vi "set Always On Top.vi"(8 "error in (no error)":errorcluster, 10 "Always On Top":bool, 11 "Actor in":refnum<class "Actor.lvclass">) -> (0 "error out":errorcluster, 3 "Actor out":refnum<class "Actor.lvclass">)   [LabVIEW 2015, in "Actor.lvclass"]
uses:
  Actor.lvclass
  Actor.lvclass/Actor.ctl
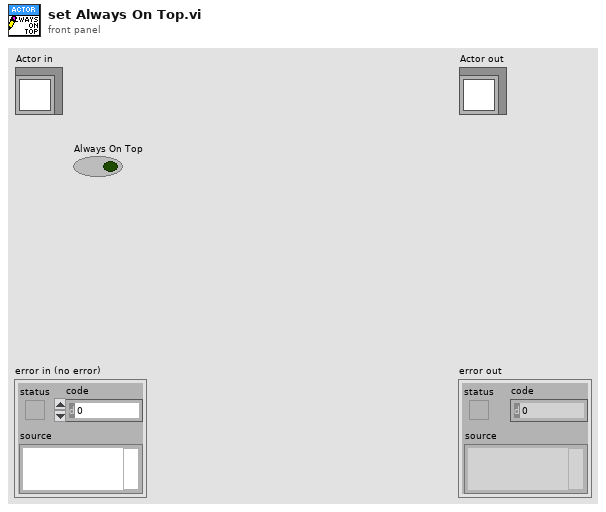
[diagram p1: front panel]
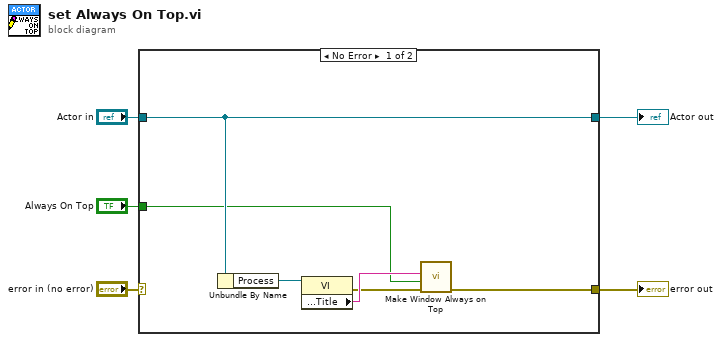
[diagram p0: block diagram]
diagram:
  n1 = case shown="No Error" "error in (no error)" {
    selector: "error in (no error)" -> [_ w12]
    tunnel: [w6 w12] -> w4
    tunnel: [w11 w13] -> w2
    tunnel: "Actor in" -> [w11 w13]
    tunnel: "Always On Top" -> [w8 _]
    frame No Error {
      n2 = Unbundle By Name(w11) -> ("Process"=w10:refnum<vi>)
      n3 = property class="VI"(reference=w10) -> (error out=w7:errorcluster, "Front Panel.Title"=w9:string)  [unwired: 1 in, 1 out]
      n4 = call "Make Window Always on Top.vi"("error in (no error)"=w7, "activate? (F)"=w8, "window name (\"\")"=w9) -> ("error out"=w6:errorcluster)  [unwired: 3 in, 1 out]
    }
    frame Error {
    }
  }
  "error out" <- w4
  "Actor out" <- w2
